vi "Acquire Every Image (Optimized Performance).vi"() -> ()   [LabVIEW 2023]
doc: "The Acquire Every Image (Optimized Performance) example shows the basics of using a ring acquisition. There are some camera restrictions to using this mode that are described in more detail in the block diagram of the VI, but it is recommended to use this method for performance-critical applications when possible."
uses:
  <vilib>/vision/driver/IMAQdx.llb/IMAQdx Acquisition Mode.ctl
  <vilib>/vision/driver/IMAQdx.llb/IMAQdx Buffer Number Mode.ctl
  <vilib>/vision/driver/NI_Vision_Acquisition_Software.lvlib
  <resource>/objmgr/imaqdx.rc
panel:
  in  "Overwrite Mode":u16(ring) items=["Get Oldest"=0, "Fail"=2, "Get Newest"=3]
  in  "Simulated Processing Delay (ms)":i32
  out "Images Missed":u32
  out "Images Behind":i32
  out "Processing Frame Rate":dbl
  in  "Number of Images":i32=10
  in  "Camera Name":refnum<k21> caption="IMAQdx Session"
  out "Buffer Number":u32
  out "Image":T1(plugin-control)
  out "Acquired Frame Rate":dbl
  in  "Stop":bool
  # "Overview: Demonstrates how to acquire continuous images using a ring acquisition, which is optimized for performance.\nRequirements: Vision Acquisition Software\nInstructions:\n1. Select the Camera Name\n2. Run the VI\n3. Increase the Simulated Processing Delay to see the effect on Images Behind and Images Missed when the acquisition loop isn't executed as quickly as the camera acquires images."
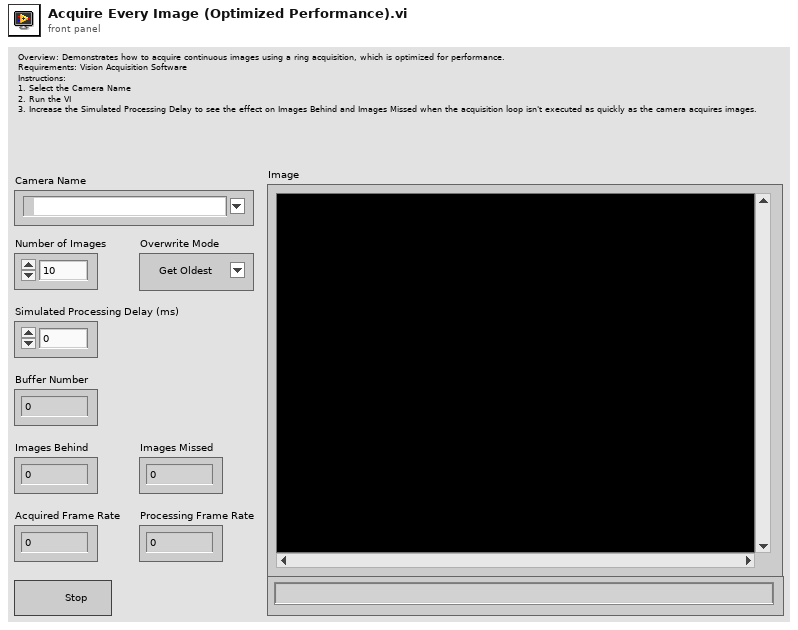
[diagram p1: front panel]
types:
  T1 = typedef "IMAQ Image.ctl" = refnum<image>
  T2 = typedef "NI_Vision_Acquisition_Software.lvlib/IMAQdx Acquisition Mode.ctl" = enum32{"One Shot", "Continuous"}
  T3 = typedef "IMAQdx.ctl" = refnum<k21>
  T4 = typedef "NI_Vision_Acquisition_Software.lvlib/IMAQdx Buffer Number Mode.ctl" = enum32{"Next", "Last", "Buffer Number", "Every", "Last New"}
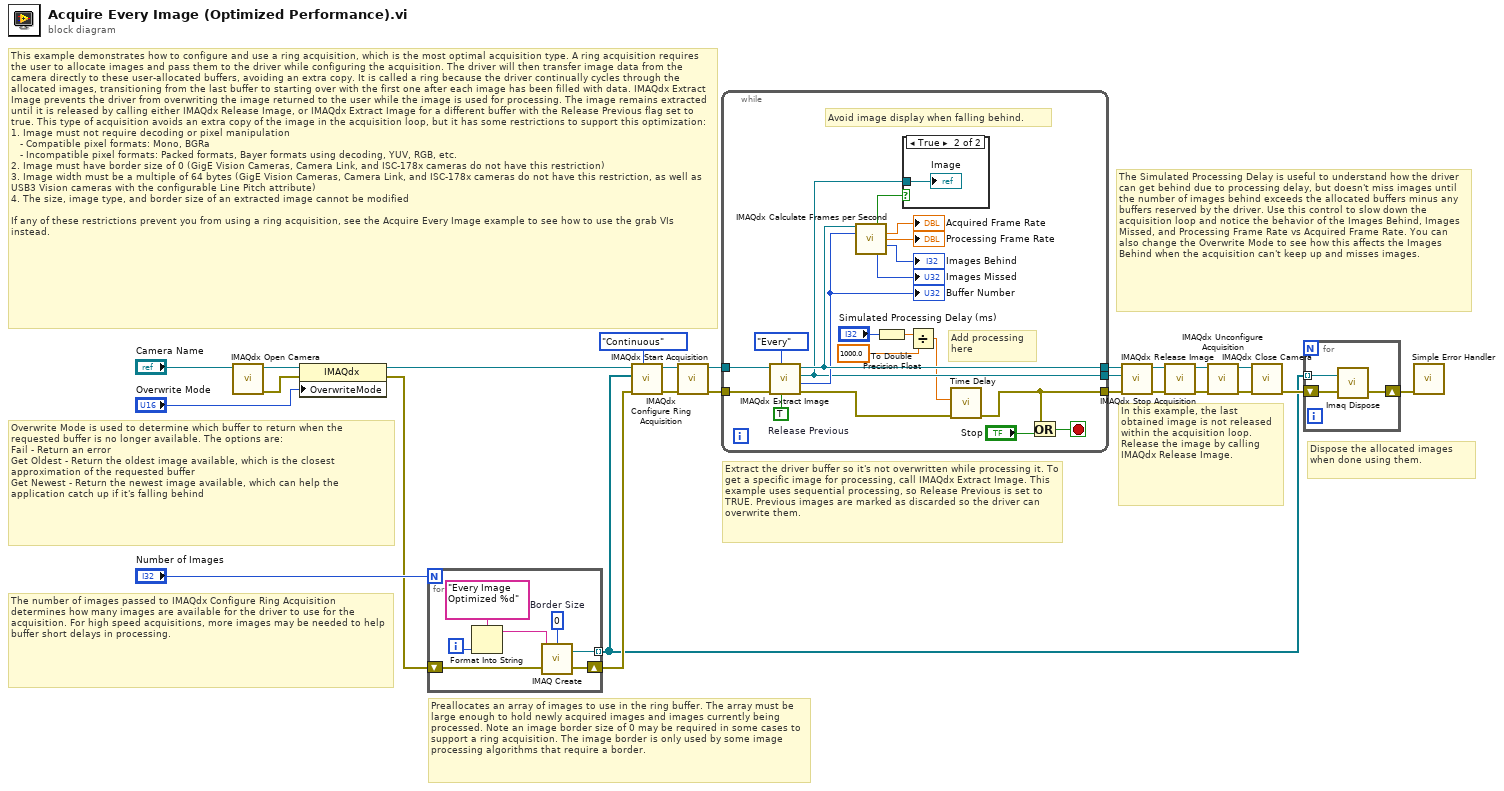
[diagram p0: block diagram]
diagram:
  # "The Simulated Processing Delay is useful to understand how the driver can get behind due to processing delay, but doesn't miss images until the number of images behind exceeds the allocated buffers minus any buffers reserved by the driver. Use this control to slow down the acquisition loop and notice the behavior of the Images Behind, Images Missed, and Processing Frame Rate vs Acquired Frame Rate. You can also change the Overwrite Mode to see how this affects the Images Behind when the acquisition can't keep up and misses images."
  # "Dispose the allocated images when done using them."
  # "The number of images passed to IMAQdx Configure Ring Acquisition determines how many images are available for the driver to use for the acquisition. For high speed acquisitions, more images may be needed to help buffer short delays in processing."
  # "Overwrite Mode is used to determine which buffer to return when the requested buffer is no longer available. The options are:\nFail - Return an error\nGet Oldest - Return the oldest image available, which is the closest approximation of the requested buffer\nGet Newest - Return the newest image available, which can help the application catch up if it's falling behind"
  # "This example demonstrates how to configure and use a ring acquisition, which is the most optimal acquisition type. A ring acquisition requires the user to allocate images and pass them to the driver while configuring the acquisition. The driver will then transfer image data from the camera directly to these user-allocated buffers, avoiding an extra copy. It is called a ring because the driver continually cycles through the allocated images, transitioning from the last buffer to starting over with the first one after each image has been filled with data. IMAQdx Extract Image prevents the driver from overwriting the image returned to the user while the image is used for processing. The image remains extracted until it is released by calling either IMAQdx Release Image, or IMAQdx Extract Image for a different buffer with the Release Previous flag set to true. This type of acquisition avoids an extra copy of the image in the acquisition loop, but it has some restrictions to support this optimization:\n1. Image must not require decoding or pixel manipulation\n   - Compatible pixel formats: Mono, BGRa\n   - Incompatible pixel formats: Packed formats, Bayer formats using decoding, YUV, RGB, etc.\n2. Image must have border size of 0 (GigE Vision Cameras, Camera Link, and ISC-178x cameras do not have this restriction)\n3. Image width must be a multiple of 64 bytes (GigE Vision Cameras, Camera Link, and ISC-178x cameras do not have this restriction, as well as USB3 Vision cameras with the configurable Line Pitch attribute)\n4. The size, image type, and border size of an extracted image cannot be modified\n\nIf any of these restrictions prevent you from using a ring acquisition, see the Acquire Every Image example to see how to use the grab VIs instead."
  # "In this example, the last obtained image is not released within the acquisition loop. Release the image by calling IMAQdx Release Image."
  # "Extract the driver buffer so it's not overwritten while processing it. To get a specific image for processing, call IMAQdx Extract Image. This example uses sequential processing, so Release Previous is set to TRUE. Previous images are marked as discarded so the driver can overwrite them."
  # "Preallocates an array of images to use in the ring buffer. The array must be large enough to hold newly acquired images and images currently being processed. Note an image border size of 0 may be required in some cases to support a ring acquisition. The image border is only used by some image processing algorithms that require a border."
  n1 = call <vilib>:"IMAQdx Open Camera.vi"("Session In"="Camera Name") -> ("error out"=w3:errorcluster, "Session Out"=w5:T3)  [unwired: 2 in, 7 out]
  n2 = property class="IMAQdx"(reference=w5, error in=w3, "OverwriteMode"="Overwrite Mode") -> (reference out=w4:T3, error out=w2:errorcluster)
  n3 = for {
    N: "Number of Images" -> [_]
    tunnel: [w31] -> w6 mode=indexing
    shift-right: [w30] -> w13
    shift-left: w2 -> [w32]
    i -> [w29]
    w26 = 0  # Border Size
    n4 = Format Into String(format string="Every Image Optimized %d" ("Image Name"), w29) -> (resulting string=w28:string)  [unwired: 2 in, 1 out]
    n5 = call "IMAQ Create"("Border Size"=w26, "Image Name"=w28, "error in (no error)"=w32) -> ("New Image"=w31:T1, "error out"=w30:errorcluster)  [unwired: 1 in, 1 out]
  }
  n6 = call <vilib>:"IMAQdx Configure Ring Acquisition.vi"("Mode"=IMAQdx_Acquisition_Mode."Continuous" ("Continuous?"), "error in"=w13, "Images"=w6, "Session In"=w4) -> ("error out"=w14:errorcluster, "Session Out"=w15:T3)  [unwired: 5 in, 1 out]
  n7 = call <vilib>:"IMAQdx Start Acquisition.vi"("error in"=w14, "Session In"=w15) -> ("error out"=w23:errorcluster, "Session Out"=w24:T3)  [unwired: 8 out]
  n8 = while {
    tunnel: [w46] -> w8
    tunnel: w23 -> [w50]
    tunnel: w24 -> [w51]
    tunnel: [w40] -> w10
    tunnel: [w42] -> w11
    stop <- w52 stop-if-true
    w47 = TRUE  # Release Previous
    # "Avoid image display when falling behind."
    # "Add processing here"
    n9 = call <vilib>:"IMAQdx Extract Image.vi"("Release Previous (true)"=w47, "Buffer Number Mode (Next)"=IMAQdx_Buffer_Number_Mode."Every" ("Buffer Number Mode"), "error in"=w50, "Session In"=w51) -> ("error out"=w41:errorcluster, "Buffer Number Out"=w45:u32, "Image Out"=w42:T1, "Session Out"=w46:T3)  [unwired: 4 in]
    "Buffer Number" <- w45
    n10 = call <vilib>:"IMAQdx Calculate Frames per Second.vi"("Session In"=w46, "Buffer Number"=w45) -> ("Update Display"=w43:bool, "Acquired Frames per Second"=→"Acquired Frame Rate":dbl, "Processed Frames per Second"=→"Processing Frame Rate":dbl, "Images Behind"=→"Images Behind":i32, "Images Missed"=→"Images Missed":u32)  [unwired: 7 in, 2 out]
    n11 = To Double Precision Float(number="Simulated Processing Delay (ms)") -> (double precision float=w33:dbl)
    n12 = case shown="True" w43 {
      tunnel: w42 -> [_ w53]
      frame False {
      }
      frame True {
        "Image" <- w53
      }
    }
    n13 = Divide(x=w33, y=1000.0) -> (x/y=w37:dbl)
    n14 = call "Time Delay"("error in (no error)"=w41, "Delay Time (s)"=w37) -> ("error out"=w40:errorcluster)  [unwired: 9 in]
    n15 = Or(x=w40, y="Stop") -> (x .or. y?=w52:bool)
  }
  n16 = call <vilib>:"IMAQdx Release Image.vi"("error in"=w10, "Image"=w11, "Session In"=w8) -> ("error out"=w9:errorcluster, "Session Out"=w7:T3)  [unwired: 7 in]
  n17 = call <vilib>:"IMAQdx Stop Acquisition.vi"("error in"=w9, "Session In"=w7) -> ("error out"=w19:errorcluster, "Session Out"=w20:T3)  [unwired: 8 out]
  n18 = call <vilib>:"IMAQdx Unconfigure Acquisition.vi"("error in"=w19, "Session In"=w20) -> ("error out"=w22:errorcluster, "Session Out"=w21:T3)  [unwired: 8 out]
  n19 = call <vilib>:"IMAQdx Close Camera.vi"("error in"=w22, "Session In"=w21) -> ("error out"=w18:errorcluster)  [unwired: 9 out]
  n20 = for {
    shift-right: [w55] -> w17
    shift-left: w18 -> [w56]
    tunnel: w6 -> [w54] mode=indexing
    n21 = call "Imaq Dispose"("Image"=w54, "error in (no error)"=w56) -> ("error out"=w55:errorcluster)  [unwired: 4 in]
  }
  n22 = call <vilib>:"Simple Error Handler.vi"("error in (no error)"=w17) -> ()  [unwired: 4 in, 5 out]
